vi "CheckRecordBitLDO.vi"(11 "Int array data from queue":u16[](array[numeric])) -> (3 "Record bit T/F":bool)   [LabVIEW 2023, in "WritingDataFile.lvlib"]
uses:
  WritingDataFile.lvlib
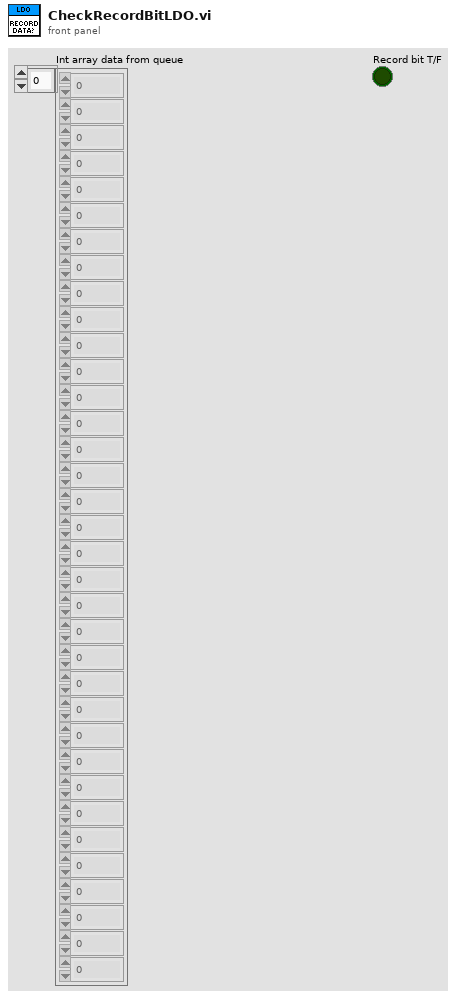
[diagram p1: front panel]
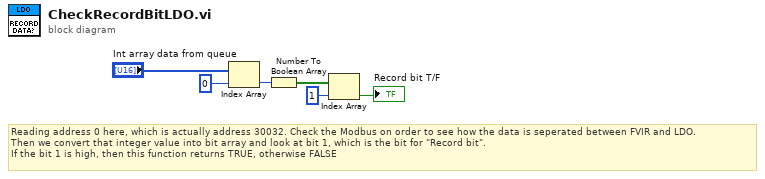
[diagram p0: block diagram]
diagram:
  # "Reading address 0 here, which is actually address 30032. Check the Modbus on order to see how the data is seperated between FVIR and LDO. \nThen we convert that integer value into bit array and look at bit 1, which is the bit for \"Record bit\". \nIf the bit 1 is high, then this function returns TRUE, otherwise FALSE"
  n1 = Index Array(array="Int array data from queue", index=0) -> (element=w2:u16)
  n2 = Number To Boolean Array(number=w2) -> (Boolean array=w3:bool[])
  n3 = Index Array(array=w3, index=1) -> (element=→"Record bit T/F":bool)
